vi "fileObjectivesRegistrationMostRecent.vi"() -> (0 "f":string)   [LabVIEW 2017]
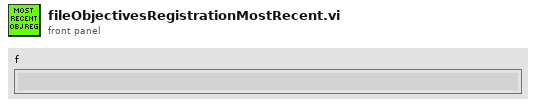
[diagram p1: front panel]
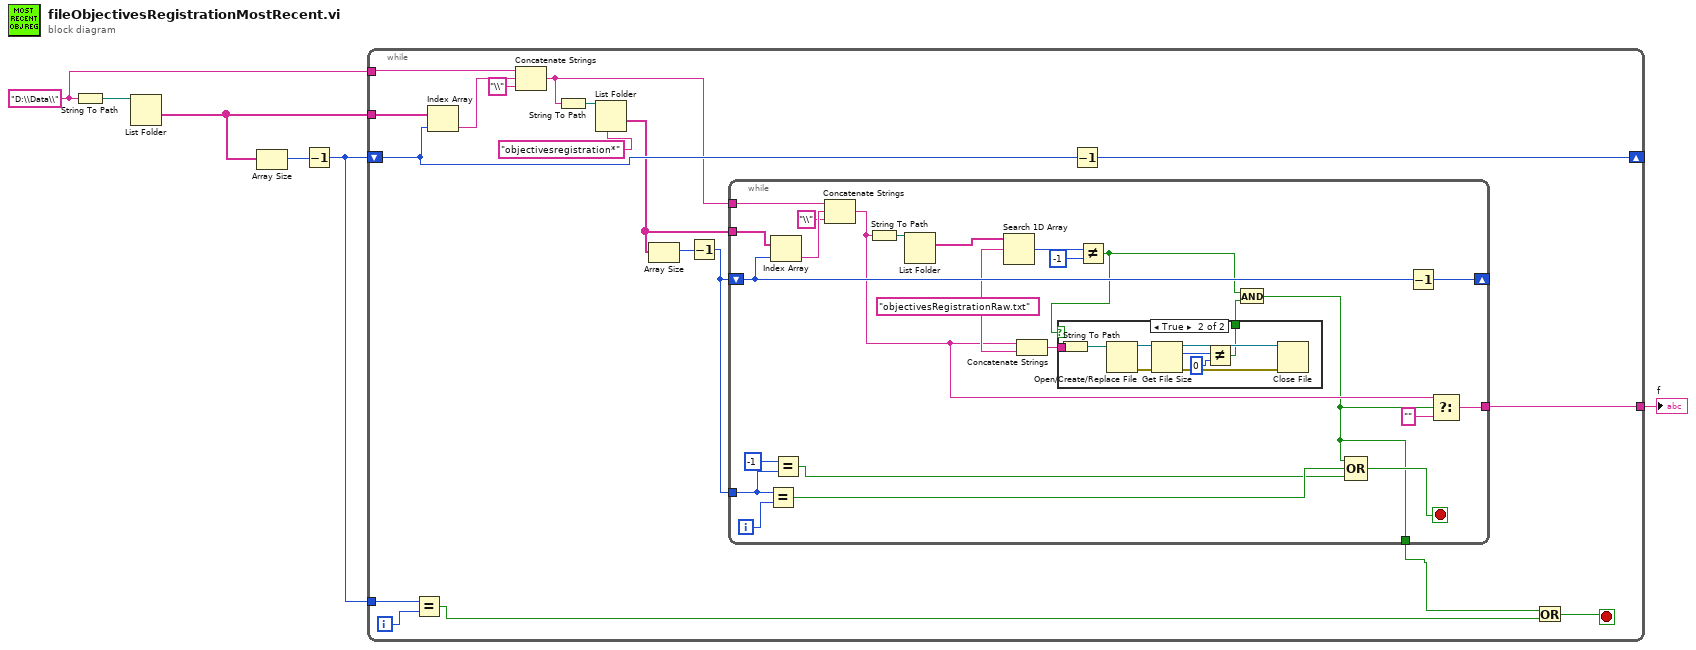
[diagram p0: block diagram]
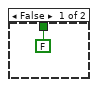
[diagram p2: hidden frame]
diagram:
  w3 = "D:\\Data\\" ("string")
  n1 = String To Path(string=w3) -> (path=w6:path)
  n2 = List Folder(path=w6) -> (folder names=w4:string[])  [unwired: 3 in, 3 out]
  n3 = Array Size(array=w4) -> (size(s)=w5:i32)
  n4 = Decrement(x=w5) -> (x-1=w2:i32)
  n5 = while {
    tunnel: w4 -> [w24]
    tunnel: w3 -> [w23]
    shift-right: [w19] -> _
    shift-left: w2 -> [w18]
    tunnel: w2 -> [w11]
    tunnel: [w9] -> w1
    i -> [w12]
    stop <- w8 stop-if-true
    n6 = Equal?(x=w11, y=w12) -> (x = y?=w10:bool)
    n7 = Index Array(array=w24, index=w18) -> (element=w22:string)
    n8 = Concatenate Strings(w23, w22, "\\" ("string")) -> (w14:string)
    n9 = String To Path(string=w14) -> (path=w20:path)
    n10 = List Folder(path=w20, pattern="objectivesregistration*") -> (folder names=w16:string[])  [unwired: 2 in, 3 out]
    n11 = Array Size(array=w16) -> (size(s)=w15:i32)
    n12 = Decrement(x=w15) -> (x-1=w13:i32)
    n13 = while {
      tunnel: w16 -> [w48]
      tunnel: w14 -> [w47]
      shift-right: [w43] -> _
      shift-left: w13 -> [w42]
      tunnel: w13 -> [w28]
      tunnel: [w32] -> w9
      tunnel: [w25] -> w7
      i -> [w36]
      stop <- w31 stop-if-true
      w38 = "objectivesRegistrationRaw.txt" ("element")
      n14 = Equal?(x=w28, y=w36) -> (x = y?=w35:bool)
      n15 = Index Array(array=w48, index=w42) -> (element=w46:string)
      n16 = Equal?(x=-1, y=w28) -> (x = y?=w26:bool)
      n17 = Concatenate Strings(w47, w46, "\\" ("string")) -> (w29:string)
      n18 = String To Path(string=w29) -> (path=w44:path)
      n19 = List Folder(path=w44) -> (filenames=w41:string[])  [unwired: 3 in, 3 out]
      n20 = Search 1D Array(1D array=w41, element=w38) -> (index of element=w40:i32)  [unwired: 1 in]
      n21 = Concatenate Strings(w29, w38) -> (w34:string)
      n22 = Not Equal?(x=w40, y=-1) -> (x != y?=w30:bool)
      n23 = case shown="True" w30 {
        tunnel: [FALSE w51] -> w37
        tunnel: w34 -> [_ w50]
        frame False {
        }
        frame True {
          n24 = String To Path(string=w50) -> (path=w58:path)
          n25 = Open/Create/Replace File(file path (use dialog)=w58) -> (refnum out=w57:refnum<file>, error out=w56:errorcluster)  [unwired: 5 in, 1 out]
          n26 = Get File Size(file=w57, error in=w56) -> (refnum out=w53:refnum<file>, size (in bytes)=w55:i64, 0:w52:errorcluster)
          n27 = Not Equal?(x=w55, y=i64 0) -> (x != y?=w51:bool)
          n28 = Close File(refnum=w53, error in=w52) -> ()  [unwired: 2 out]
        }
      }
      n29 = And(x=w30, y=w37) -> (x .and. y?=w25:bool)
      n30 = Compound Arithmetic op=OR(w25, w35, w26) -> (w31:bool)
      n31 = Decrement(x=w42) -> (x-1=w43:i32)
      n32 = Select(t=w29, s=w25, f="") -> (s? t:f=w32:string)
    }
    n33 = Decrement(x=w18) -> (x-1=w19:i32)
    n34 = Or(x=w7, y=w10) -> (x .or. y?=w8:bool)
  }
  "f" <- w1
